vi "Calibrate Array.vi"(11 "Array In":dbl[][](array[numeric])) -> (1 "b values":dbl[](array[numeric]), 2 "m values":dbl[](array[numeric]), 3 "R^2 values":dbl[](array[numeric]), 5 "String Array":string[][](array[string]))   [LabVIEW 2020]
uses:
  <vilib>/Analysis/6fits.llb/Curve Fitting Criteria.ctl
  <vilib>/Analysis/NI_AALPro.lvlib
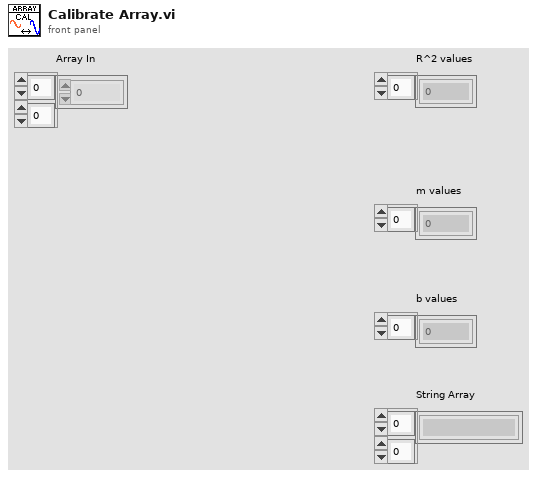
[diagram p1: front panel]
types:
  T1 = typedef "NI_AALPro.lvlib/Curve Fitting Criteria.ctl" = u16
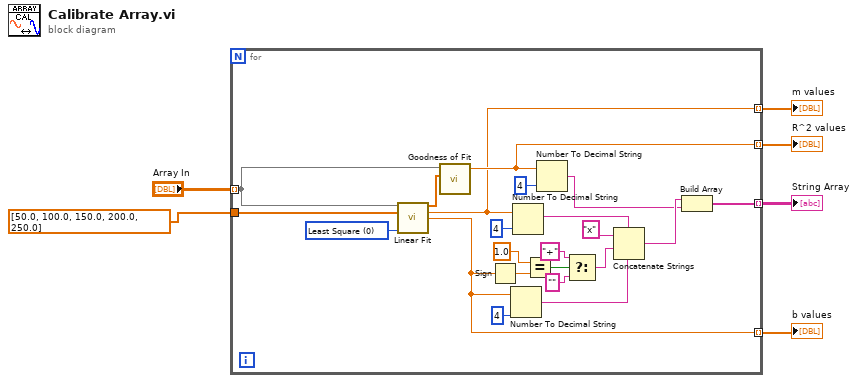
[diagram p0: block diagram]
diagram:
  n1 = for {
    tunnel: "Array In" -> [w26] mode=indexing
    tunnel: dbl[] [50.0, 100.0, 150.0, 200.0, 250.0] -> [w27]
    tunnel: [w10] -> w3 mode=indexing
    tunnel: [w9] -> w4 mode=indexing
    tunnel: [w8] -> w5 mode=indexing
    tunnel: [w7] -> w6 mode=indexing
    w28 = T1 0 items=["Least Square", "Least Absolute Residual", "Bisquare"] ("method")
    n2 = call <vilib>:"Linear Fit.vi"("Y"=w26, "X"=w27, "method"=w28) -> ("Best Linear Fit"=w25:dbl[], "slope"=w8:dbl, "intercept"=w7:dbl)  [unwired: 8 in, 2 out]
    n3 = call <vilib>:"Goodness of Fit.vi"("Best Fit"=w25, "Y"=w26) -> ("R-square"=w9:dbl)  [unwired: 6 in, 3 out]
    n4 = Sign(1:w7) -> (0:w18:dbl)
    n5 = Number To Decimal String(number=w7, width (-)=i16 4) -> (decimal integer string=w19:string)
    n6 = Number To Decimal String(number=w8, width (-)=i16 4) -> (decimal integer string=w20:string)
    n7 = Equal?(x=1.0, y=w18) -> (x = y?=w16:bool)
    n8 = Number To Decimal String(number=w9, width (-)=i16 4) -> (decimal integer string=w11:string)
    n9 = Select(t="+" ("string"), s=w16, f="" ("string")) -> (s? t:f=w13:string)
    n10 = Concatenate Strings(w20, "x" ("string"), w13, w19) -> (w12:string)
    n11 = Build Array(w12, w11) -> (w10:string[])
  }
  "b values" <- w6
  "m values" <- w5
  "R^2 values" <- w4
  "String Array" <- w3
